vi "Release.vi"(8 "error in (no error)":errorcluster, 11 "SingleA in":refnum<class "SingleA.lvclass">) -> (0 "error out":errorcluster, 3 "SingleA out":refnum<class "SingleA.lvclass">)   [LabVIEW 2020, in "SingleA.lvclass"]
uses:
  SingleA.lvclass
  Singleton/Singleton.lvclass
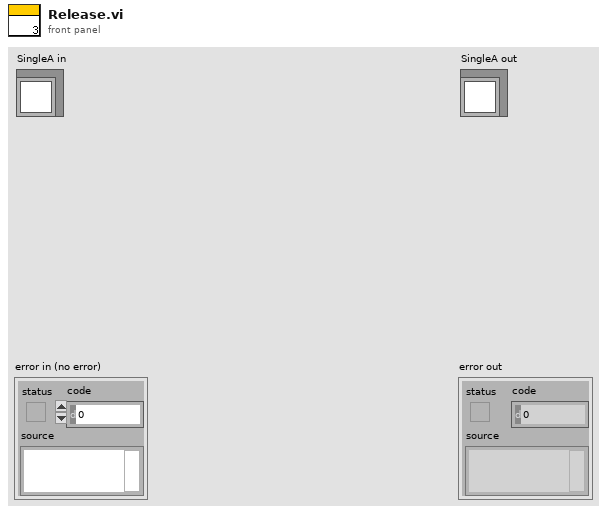
[diagram p1: front panel]
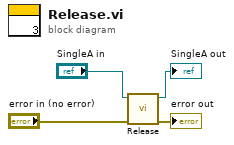
[diagram p0: block diagram]
diagram:
  n1 = call-parent "Release.vi"("error in (no error)"="error in (no error)", "Singleton in"="SingleA in") -> ("error out"=→"error out":errorcluster, "Singleton out"=→"SingleA out":refnum<class "SingleA.lvclass">)  [unwired: 8 in]
